vi "interface.vi"() -> ()   [LabVIEW 2023]
uses:
  <vilib>/Instr/_visa.llb/VISA Configure Serial Port (Instr).vi
  <vilib>/ptbypt/NI_PtbyPt.lvlib
panel:
  in  "Tab Control":enum32{"Electrocardiograph", "Settings"}(tab)
  out "ECG":u8(graph)
  out "BPM":dbl(graph)
  out "BPM":dbl format="%#.0f"
  in  "Sample Rate (S/s)":u16(ring) items=["50", "75", "100", "200"]
  in  "Iniciar":bool
  in  "stop":bool
  out "R Wave Detection":bool
  in  "Arduino Mode":bool
  out "Manual":bool
  out "Automatic":bool
  out "Defibrillator":bool
  out "Pacemaker":bool
  out "Atropine":bool
  out "Propranolol 2":bool
  out "String":string
  in  "Defibrillator 2":bool
  in  "Atropine 2":bool
  in  "Pacemaker 2":bool
  in  "Save":bool
  in  "Propranolol 3":bool
  in  "Clear":bool
  out "Array":string[](array[string])
  in  "VISA resource name":refnum<visa-resource-name>="COM4"
  in  "error in (no error)":errorcluster
  out "error out":errorcluster
  in  "Upper Threshold":dbl=200.0
  in  "Lower Threshold":dbl=120.0
  in  "stop 2":bool
  # "Manual Mode"
  # "BPM"
  # "Propanolol"
  # "Atropine"
  # "Pacemaker"
  # "Defibrillator"
  # "Defibrillator Activation Time"
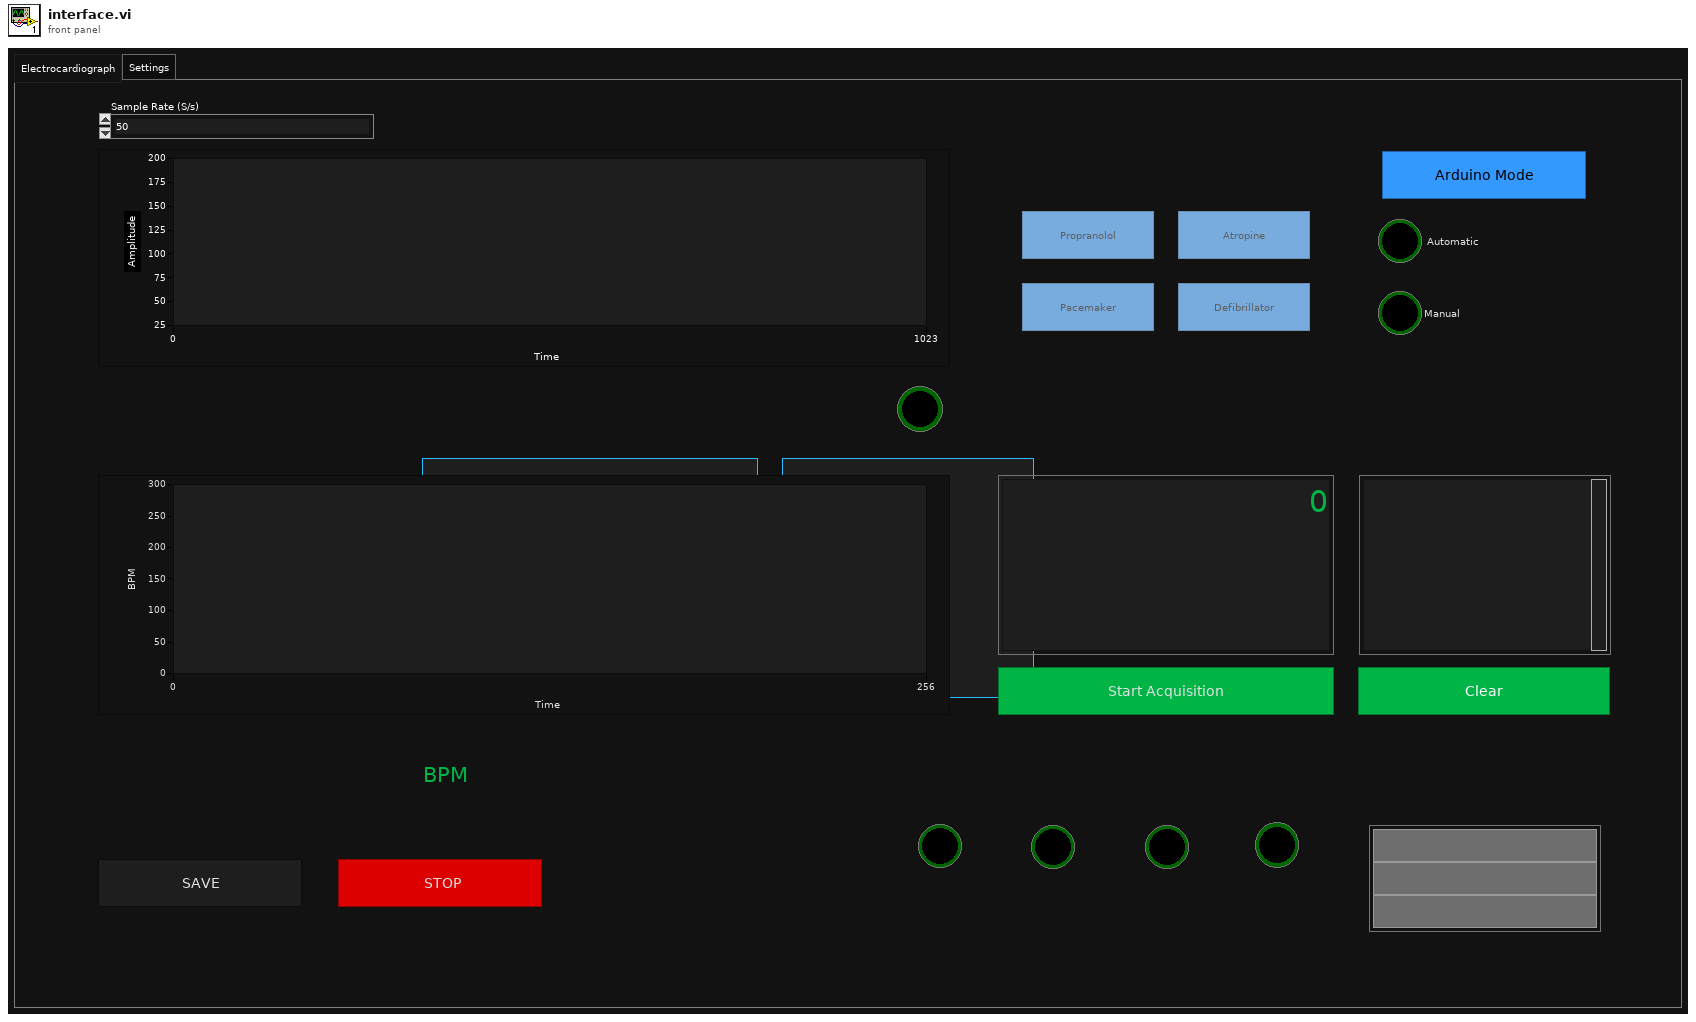
[diagram p1: front panel]
types:
  T1 = enum8{"Enabled", "Disabled", "Disabled and Grayed Out"}
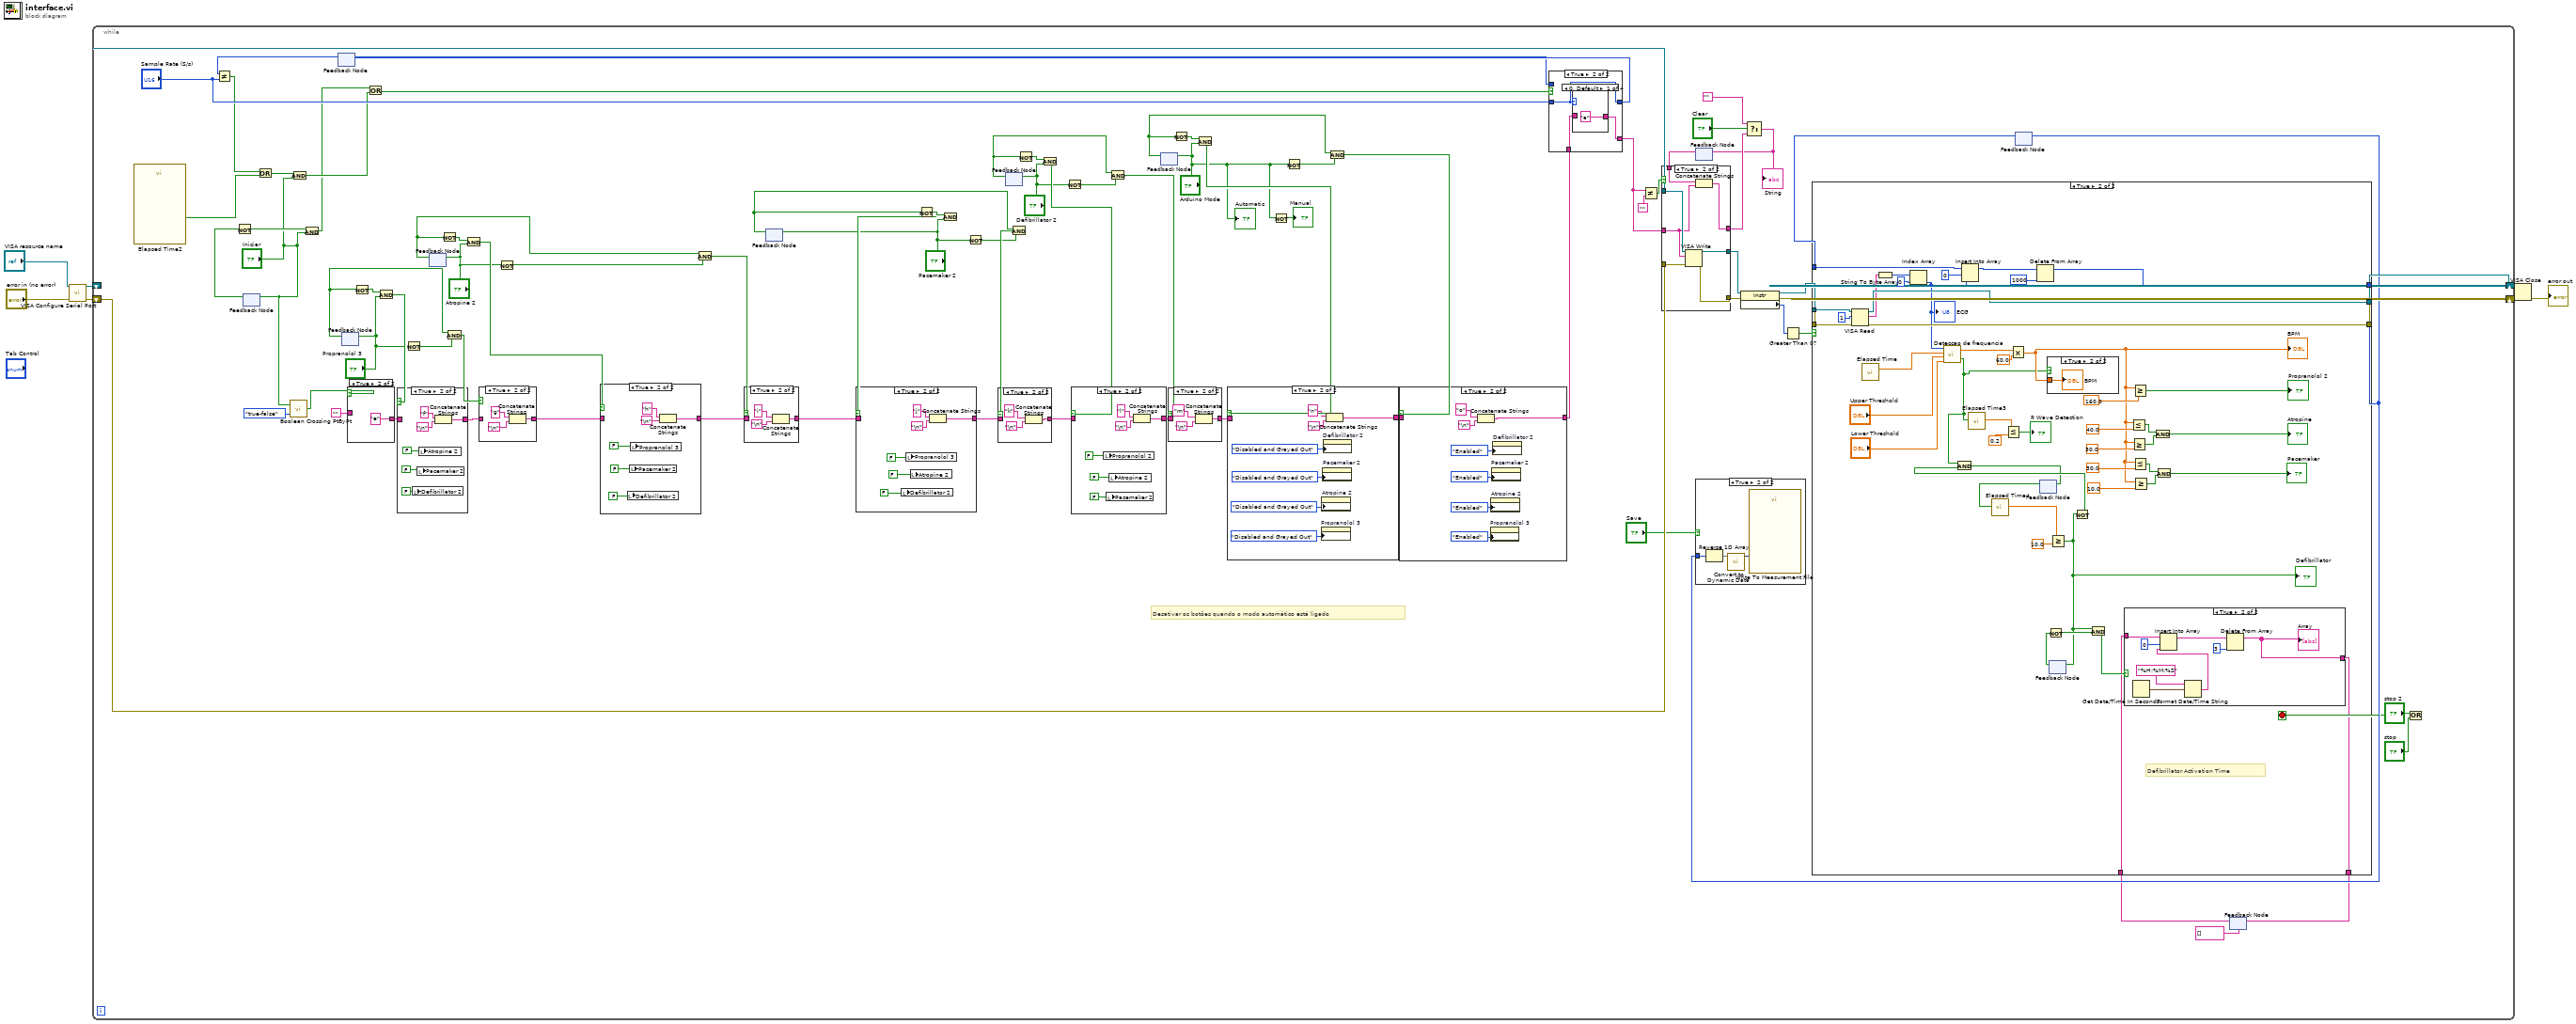
[diagram p0: block diagram]
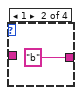
[diagram p15: hidden frame]
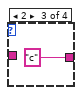
[diagram p16: hidden frame]
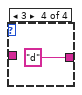
[diagram p17: hidden frame]
diagram:
  n1 = call-poly "VISA Configure Serial Port"("VISA resource name"="VISA resource name", "error in (no error)"="error in (no error)") -> ("VISA resource name out"=w5:refnum<visa-resource-name>, "error out"=w4:errorcluster)  [unwired: 12 in]
  n2 = while {
    shift-right: [w87] -> w3
    shift-left: w5 -> [w85]
    shift-right: [w86] -> w2
    shift-left: w4 -> [w84]
    stop <- w61 stop-if-true
    # "Desativar os botões quando o modo automático está ligado"
    n3 = call "Elapsed Time2"() -> ("Time has Elapsed"=w72:bool)  [unwired: 12 in, 7 out]
    n4 = feedback-in #1("Iniciar") -> ()
    n5 = feedback #1() -> (w65:bool)  [unwired: 1 in]
    n6 = Not(x=w65) -> (.not. x?=w66:bool)
    n7 = call <vilib>:"Boolean Crossing PtByPt.vi"("direction"=enum16{"either", "false-true", "true-false"}."true-false", "input"="Iniciar") -> ("crossing"=w22:bool)  [unwired: 1 in]
    n8 = And(x=w66, y="Iniciar") -> (x .and. y?=w64:bool)
    n9 = feedback #2() -> (w76:u16)  [unwired: 1 in]
    n10 = Not Equal?(x=w76, y="Sample Rate (S/s)") -> (x != y?=w69:bool)
    n11 = Or(x=w69, y=w72) -> (x .or. y?=w71:bool)
    n12 = And(x=w71, y="Iniciar") -> (x .and. y?=w67:bool)
    n13 = feedback-in #3("Propranolol 3") -> ()
    n14 = feedback #3() -> (w57:bool)  [unwired: 1 in]
    n15 = case shown="True" w22 {
      tunnel: [w152 "e"] -> w42
      tunnel: "" -> [w152 _]
      frame False {
      }
      frame True {
      }
    }
    n16 = Not(x=w57) -> (.not. x?=w60:bool)
    n17 = Or(x=w64, y=w67) -> (x .or. y?=w68:bool)
    n18 = And(x=w60, y="Propranolol 3") -> (x .and. y?=w59:bool)
    n19 = case shown="True" w59 {
      tunnel: w42 -> [w145 _]
      tunnel: [w145 w151] -> w41
      frame False {
      }
      frame True {
        n20 = local write "Defibrillator 2"(FALSE) -> ()
        n21 = local write "Pacemaker 2"(FALSE) -> ()
        n22 = local write "Atropine 2"(FALSE) -> ()
        n23 = Concatenate Strings("f", "\n") -> (w151:string)
      }
    }
    n24 = Not(x="Propranolol 3") -> (.not. x?=w56:bool)
    n25 = feedback #4() -> (w52:bool)  [unwired: 1 in]
    n26 = feedback-in #4("Atropine 2") -> ()
    n27 = Not(x=w52) -> (.not. x?=w55:bool)
    n28 = And(x=w57, y=w56) -> (x .and. y?=w58:bool)
    n29 = And(x=w55, y="Atropine 2") -> (x .and. y?=w54:bool)
    n30 = case shown="True" w58 {
      tunnel: w41 -> [w141 _]
      tunnel: [w141 w144] -> w40
      frame False {
      }
      frame True {
        n31 = Concatenate Strings("g", "\n") -> (w144:string)
      }
    }
    n32 = Not(x="Atropine 2") -> (.not. x?=w51:bool)
    n33 = case shown="True" w54 {
      tunnel: w40 -> [w134 _]
      tunnel: [w134 w140] -> w39
      frame False {
      }
      frame True {
        n34 = local write "Defibrillator 2"(FALSE) -> ()
        n35 = local write "Pacemaker 2"(FALSE) -> ()
        n36 = local write "Propranolol 3"(FALSE) -> ()
        n37 = Concatenate Strings("h", "\n") -> (w140:string)
      }
    }
    n38 = And(x=w52, y=w51) -> (x .and. y?=w53:bool)
    n39 = case shown="True" w53 {
      tunnel: w39 -> [w130 _]
      tunnel: [w130 w133] -> w38
      frame False {
      }
      frame True {
        n40 = Concatenate Strings("i", "\n") -> (w133:string)
      }
    }
    n41 = feedback #5() -> (w47:bool)  [unwired: 1 in]
    n42 = feedback-in #5("Pacemaker 2") -> ()
    n43 = Not(x=w47) -> (.not. x?=w50:bool)
    n44 = And(x=w50, y="Pacemaker 2") -> (x .and. y?=w49:bool)
    n45 = case shown="True" w49 {
      tunnel: w38 -> [w123 _]
      tunnel: [w123 w129] -> w37
      frame False {
      }
      frame True {
        n46 = local write "Defibrillator 2"(FALSE) -> ()
        n47 = local write "Propranolol 3"(FALSE) -> ()
        n48 = local write "Atropine 2"(FALSE) -> ()
        n49 = Concatenate Strings("j", "\n") -> (w129:string)
      }
    }
    n50 = Not(x="Pacemaker 2") -> (.not. x?=w46:bool)
    n51 = feedback #6() -> (w28:bool)  [unwired: 1 in]
    n52 = feedback-in #6("Defibrillator 2") -> ()
    n53 = And(x=w47, y=w46) -> (x .and. y?=w48:bool)
    n54 = case shown="True" w48 {
      tunnel: w37 -> [w119 _]
      tunnel: [w119 w122] -> w24
      frame False {
      }
      frame True {
        n55 = Concatenate Strings("k", "\n") -> (w122:string)
      }
    }
    n56 = Not(x=w28) -> (.not. x?=w31:bool)
    n57 = And(x=w31, y="Defibrillator 2") -> (x .and. y?=w30:bool)
    n58 = Not(x="Defibrillator 2") -> (.not. x?=w27:bool)
    n59 = case shown="True" w30 {
      tunnel: w24 -> [w112 _]
      tunnel: [w112 w118] -> w25
      frame False {
      }
      frame True {
        n60 = local write "Propranolol 2"(FALSE) -> ()
        n61 = local write "Pacemaker 2"(FALSE) -> ()
        n62 = local write "Atropine 2"(FALSE) -> ()
        n63 = Concatenate Strings("l", "\n") -> (w118:string)
      }
    }
    n64 = And(x=w28, y=w27) -> (x .and. y?=w29:bool)
    n65 = feedback #7() -> (w19:bool)  [unwired: 1 in]
    n66 = feedback-in #7("Arduino Mode") -> ()
    n67 = case shown="True" w29 {
      tunnel: w25 -> [w108 _]
      tunnel: [w108 w111] -> w16
      frame False {
      }
      frame True {
        n68 = Concatenate Strings("m", "\n") -> (w111:string)
      }
    }
    n69 = Not(x=w19) -> (.not. x?=w20:bool)
    n70 = And(x=w20, y="Arduino Mode") -> (x .and. y?=w13:bool)
    n71 = case shown="True" w13 {
      tunnel: [w100 w107] -> w17
      tunnel: w16 -> [w100 _]
      frame False {
      }
      frame True {
        n72 = property on="Propranolol 3" class="Bool (strict)"("DisabledEnum"=T1."Disabled and Grayed Out" ("Disabled")) -> ()  [unwired: 2 in, 2 out]
        n73 = property on="Atropine 2" class="Bool (strict)"("DisabledEnum"=T1."Disabled and Grayed Out" ("Disabled")) -> ()  [unwired: 2 in, 2 out]
        n74 = property on="Pacemaker 2" class="Bool (strict)"("DisabledEnum"=T1."Disabled and Grayed Out" ("Disabled")) -> ()  [unwired: 2 in, 2 out]
        n75 = property on="Defibrillator 2" class="Bool (strict)"("DisabledEnum"=T1."Disabled and Grayed Out" ("Disabled")) -> ()  [unwired: 2 in, 2 out]
        n76 = Concatenate Strings("n", "\n") -> (w107:string)
      }
    }
    n77 = Not(x="Arduino Mode") -> (.not. x?=→"Manual":bool)
    n78 = Not(x="Arduino Mode") -> (.not. x?=w18:bool)
    n79 = And(x=w19, y=w18) -> (x .and. y?=w14:bool)
    n80 = case shown="True" w14 {
      tunnel: w17 -> [w92 _]
      tunnel: [w92 w99] -> w15
      frame False {
      }
      frame True {
        n81 = Concatenate Strings("o", "\n") -> (w99:string)
        n82 = property on="Propranolol 3" class="Bool (strict)"("DisabledEnum"=T1."Enabled" ("Disabled")) -> ()  [unwired: 2 in, 2 out]
        n83 = property on="Atropine 2" class="Bool (strict)"("DisabledEnum"=T1."Enabled" ("Disabled")) -> ()  [unwired: 2 in, 2 out]
        n84 = property on="Pacemaker 2" class="Bool (strict)"("DisabledEnum"=T1."Enabled" ("Disabled")) -> ()  [unwired: 2 in, 2 out]
        n85 = property on="Defibrillator 2" class="Bool (strict)"("DisabledEnum"=T1."Enabled" ("Disabled")) -> ()  [unwired: 2 in, 2 out]
      }
    }
    n86 = case shown="True" w68 {
      tunnel: "Sample Rate (S/s)" -> [w158 w160]
      tunnel: [w157 w161] -> w79
      tunnel: [w158 w160] -> w77
      tunnel: w76 -> [_ _]
      tunnel: w15 -> [w157 w159]
      frame False {
      }
      frame True {
        n87 = case shown="0, Default" w160 {
          tunnel: ["a" "b" "c" "d"] -> w161
          tunnel: w159 -> [_ _ _ _]
          frame 0, Default {
          }
          frame 1 {
          }
          frame 2 {
          }
          frame 3 {
          }
        }
      }
    }
    n88 = feedback-in #2(w77) -> ()
    n89 = Not Equal?(x=w79, y="") -> (x != y?=w81:bool)
    n90 = feedback #8() -> (w36:string)  [unwired: 1 in]
    n91 = case shown="True" w81 {
      tunnel: w85 -> [w168 w173]
      tunnel: w84 -> [w167 w172]
      tunnel: [w168 w175] -> w83
      tunnel: [w167 w174] -> w82
      tunnel: w79 -> [_ w171]
      tunnel: [w166 w170] -> w33
      tunnel: w36 -> [w166 w169]
      frame False {
      }
      frame True {
        n92 = VISA Write(VISA resource name=w173, write buffer=w171, error in (no error)=w172) -> (VISA resource name out=w175:refnum<visa-resource-name>, error out=w174:errorcluster)  [unwired: 1 out]
        n93 = Concatenate Strings(w169, w171) -> (w170:string)
      }
    }
    n94 = property class="Instr"(reference=w83, error in=w82) -> (reference out=w89:refnum<visa-resource-name>, error out=w88:errorcluster, "Serial Settings:Number of Bytes at Serial Port"=w91:u32)
    n95 = Select(t="", s="Clear", f=w33) -> (s? t:f=w32:string)
    "String" <- w32
    n96 = feedback-in #8(w32) -> ()
    n97 = Greater Than 0?(x=w91) -> (x > 0?=w90:bool)
    n98 = feedback #9() -> (w75:u8[])  [unwired: 1 in]
    n99 = feedback #10(string[] []) -> (w9:string[])
    n100 = case shown="True" w90 {
      tunnel: w89 -> [w179 w225]
      tunnel: w88 -> [w178 w226]
      tunnel: [w179 w223] -> w87
      tunnel: [w178 w222] -> w86
      tunnel: w75 -> [w177 w218]
      tunnel: [w177 w215] -> w74
      tunnel: w9 -> [w176 w180]
      tunnel: [w176 w181] -> w8
      frame False {
      }
      frame True {
        # "Defibrillator Activation Time"
        n101 = VISA Read(VISA resource name=w225, byte count=u32 1, error in (no error)=w226) -> (VISA resource name out=w223:refnum<visa-resource-name>, read buffer=w219:string, error out=w222:errorcluster)  [unwired: 1 out]
        n102 = call "Elapsed Time"() -> ("Elapsed Time (s)"=w212:dbl)  [unwired: 12 in, 7 out]
        n103 = String To Byte Array(string=w219) -> (unsigned byte array=w221:u8[])
        n104 = Index Array(array=w221, index=0) -> (element=w213:u8)
        "ECG" <- w213
        n105 = call "Deteccao de frequencia.vi"("Limiar inferior de deteccao"="Lower Threshold", "Limiar superior de deteccao"="Upper Threshold", "Tempo (s)"=w212, "Medida do sinal"=w213) -> ("Deteccao de limiar"=w193:bool, "Frequencia (Hz)"=w211:dbl)
        n106 = Insert Into Array "Insert Into Array"(array=w218, index=0, new element=w213) -> (w216:u8[])
        n107 = call "Elapsed Time3"("Reset"=w193) -> ("Elapsed Time (s)"=w206:dbl)  [unwired: 11 in, 7 out]
        n108 = Less Or Equal?(x=w206, y=0.2) -> (x <= y?=→"R Wave Detection":bool)
        n109 = Multiply(x=w211, y=60.0) -> (x*y=w196:dbl)
        "BPM" <- w196
        n110 = Delete From Array "Delete From Array"(array=w216, index=1000) -> (array with subset deleted=w215:u8[])  [unwired: 1 in, 1 out]
        n111 = feedback #11() -> (w190:bool)  [unwired: 1 in]
        n112 = call "Elapsed Time4"("Reset"=w190) -> ("Elapsed Time (s)"=w195:dbl)  [unwired: 11 in, 7 out]
        n113 = case shown="True" w193 {
          tunnel: w196 -> [_ w236]
          frame False {
          }
          frame True {
            "BPM" <- w236
          }
        }
        n114 = feedback #12() -> (w184:bool)  [unwired: 1 in]
        n115 = Not(x=w184) -> (.not. x?=w183:bool)
        n116 = Greater Or Equal?(x=w195, y=10.0) -> (x >= y?=w182:bool)
        "Defibrillator" <- w182
        n117 = feedback-in #12(w182) -> ()
        n118 = Not(x=w182) -> (.not. x?=w192:bool)
        n119 = And(x=w193, y=w192) -> (x .and. y?=w191:bool)
        n120 = feedback-in #11(w191) -> ()
        n121 = And(x=w182, y=w183) -> (x .and. y?=w185:bool)
        n122 = case shown="True" w185 {
          tunnel: [w227 w230] -> w181
          tunnel: w180 -> [w227 w234]
          frame False {
          }
          frame True {
            n123 = Get Date/Time In Seconds() -> (seconds since 1Jan1904=w233:timestamp)
            n124 = Format Date/Time String(time format string (%c)="%H:%M:%S", seconds (now)=w233) -> (date/time string=w231:string)  [unwired: 1 in]
            n125 = Insert Into Array(array=w234, index=0, new element=w231) -> (w229:string[])
            n126 = Delete From Array(array=w229, index=3) -> (array with subset deleted=w230:string[])  [unwired: 1 in, 1 out]
            "Array" <- w230
          }
        }
        n127 = Less Or Equal?(x=w196, y=40.0) -> (x <= y?=w203:bool)
        n128 = Greater Or Equal?(x=w196, y=30.0) -> (x >= y?=w202:bool)
        n129 = Greater Or Equal?(x=w196, y=160.0) -> (x >= y?=→"Propranolol 2":bool)
        n130 = Less Or Equal?(x=w196, y=30.0) -> (x <= y?=w199:bool)
        n131 = Greater Or Equal?(x=w196, y=10.0) -> (x >= y?=w200:bool)
        n132 = And(x=w203, y=w202) -> (x .and. y?=→"Atropine":bool)
        n133 = And(x=w199, y=w200) -> (x .and. y?=→"Pacemaker":bool)
      }
    }
    n134 = case shown="True" "Save" {
      tunnel: w74 -> [_ w156]
      frame False {
      }
      frame True {
        n135 = Reverse 1D Array(array=w156) -> (reversed array=w155:u8[])
        n136 = call "Convert to Dynamic Data"("Array"=w155) -> ("Dynamic Data Type"=w154:dynamicdata)  [unwired: 3 in]
        n137 = call "Write To Measurement File"("Signals"=w154) -> ()  [unwired: 16 in, 3 out]
      }
    }
    n138 = feedback-in #9(w74) -> ()
    n139 = feedback-in #10(w8) -> ()
    n140 = Or(x="stop 2", y="stop") -> (x .or. y?=w61:bool)
    "Automatic" <- "Arduino Mode"
  }
  n141 = VISA Close(VISA resource name=w3, error in (no error)=w2) -> (error out=→"error out":errorcluster)
